vi "Handle Message.vi"(8 "error in (no error)":errorcluster, 10 "Message":refnum<class "~Message.lvclass">, 11 "Zero Timeout Message Handler in":refnum<class "Zero Timeout Message Handler.lvclass">) -> (0 "error out":errorcluster, 3 "Zero Timeout Message Handler out":refnum<class "Zero Timeout Message Handler.lvclass">)   [LabVIEW 2024, in "Zero Timeout Message Handler.lvlib" / "Zero Timeout Message Handler.lvclass"]
uses:
  Zero Timeout Message Handler.lvclass
  ~Message/~Message.lvclass
  Zero Timeout Message Handler.lvclass/Zero Timeout Message Handler.ctl
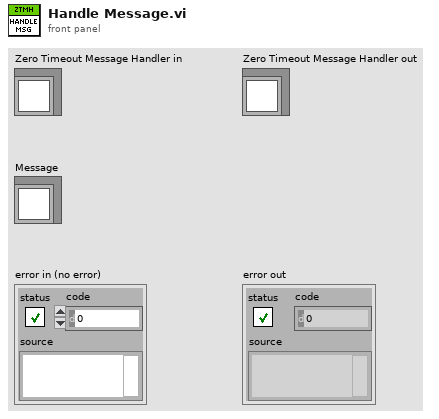
[diagram p1: front panel]
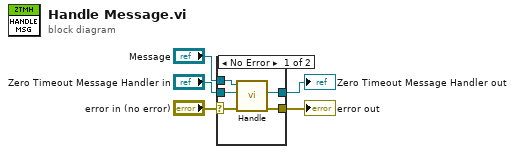
[diagram p0: block diagram]
diagram:
  n1 = case shown="No Error" "error in (no error)" {
    selector: "error in (no error)" -> [w7 w12]
    tunnel: [w6 w12] -> w4
    tunnel: [w8 w11] -> w2
    tunnel: "Zero Timeout Message Handler in" -> [w9 w11]
    tunnel: "Message" -> [w10 _]
    frame No Error {
      n2 = call-dynamic "Handle.vi"("error in (no error)"=w7, "Zero Timeout Message Handler in"=w9, "Message in"=w10) -> ("error out"=w6:errorcluster, "Zero Timeout Message Handler out"=w8:refnum<class "Zero Timeout Message Handler.lvclass">)  [unwired: 7 in]
    }
    frame Error {
    }
  }
  "error out" <- w4
  "Zero Timeout Message Handler out" <- w2
